vi "Bitmap File Writer.vi"   [LabVIEW 2018]
types:
  T1 = enum16{"open", "replace", "create", "open or create", "replace or create", "replace or create with confirmation"}
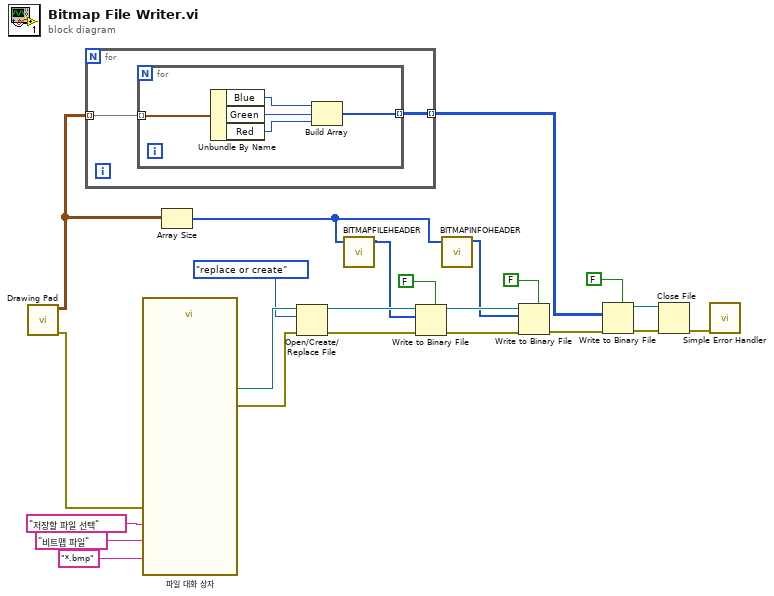
[diagram p0: block diagram]
diagram:
  n1 = call "Drawing Pad.vi"() -> ("에러 출력"=w20:errorcluster, "이미지 데이터"=w9:cluster{"Red":u8, "Green":u8, "Blue":u8}[][])  [unwired: 10 in]
  n2 = for {
    tunnel: w9 -> [w25] mode=indexing
    tunnel: [w24] -> w4 mode=indexing
    n3 = for {
      tunnel: w25 -> [w30] mode=indexing
      tunnel: [w26] -> w24 mode=indexing
      n4 = Unbundle By Name(w30) -> ("Blue"=w29:u8, "Green"=w28:u8, "Red"=w27:u8)
      n5 = Build Array(w29, w28, w27) -> (w26:u8[])
    }
  }
  n6 = call "파일 대화 상자"("prompt"="저장할 파일 선택", "error in"=w20, "pattern (all files)"="*.bmp", "pattern label"="비트맵 파일") -> ("selected path"=w18:path, "error out"=w19:errorcluster)  [unwired: 8 in, 2 out]
  n7 = Array Size(array=w9) -> (size(s)=w1:i32[])
  n8 = Open/Create/Replace File(file path (use dialog)=w18, error in=w19, operation (0:open)=T1."replace or create" ("동작(0:open)")) -> (refnum out=w14:refnum<file>, error out=w12:errorcluster)  [unwired: 3 in, 1 out]
  n9 = call "BITMAPFILEHEADER.vi"("이미지 차원"=w1) -> ("비트맵 파일 헤더"=w2:u8[])  [unwired: 10 in]
  n10 = Write to Binary File(file (use dialog)=w14, data=w2, error in=w12, 5:FALSE ("배열 또는 문자열 크기를 앞에 추가? (참)")) -> (refnum out=w13:refnum<file>, error out=w11:errorcluster)  [unwired: 2 in, 1 out]
  n11 = call "BITMAPINFOHEADER.vi"("이미지 차원"=w1) -> ("비트맵 파일 헤더"=w10:u8[])  [unwired: 10 in]
  n12 = Write to Binary File(file (use dialog)=w13, data=w10, error in=w11, 5:FALSE ("배열 또는 문자열 크기를 앞에 추가? (참)")) -> (error out=w3:errorcluster)  [unwired: 2 in, 2 out]
  n13 = Write to Binary File(data=w4, error in=w3, 5:FALSE ("배열 또는 문자열 크기를 앞에 추가? (참)")) -> (refnum out=w6:refnum<file>, error out=w7:errorcluster)  [unwired: 3 in, 1 out]
  n14 = Close File(refnum=w6, error in=w7) -> (error out=w5:errorcluster)  [unwired: 1 out]
  n15 = call <vilib>:"Simple Error Handler.vi"("error in (no error)"=w5) -> ()  [unwired: 4 in, 5 out]
